vi "PathPlanner_ConstraintsZone_IsWithinZone.vi"(9 "T":dbl, 11 "ConstraintsZone":T1) -> (3 "WithinZone":bool)   [LabVIEW 2019, in "PathPlanner24.lvlib"]
doc: "Get if a given waypoint relative position is within this zone\n \nInputs:\n -- ConstraintsZone -- cluster -- data structure containing zone definition. \n -- t - double - Waypoint relative position\n\nOutputs:\n -- WithinZone - boolean - True if given position is within this zone"
uses:
  PathPlanner24.lvlib
  TypeDef/PathPlannerConstraintsZone.ctl
  TypeDef/PathPlannerPathConstraints.ctl
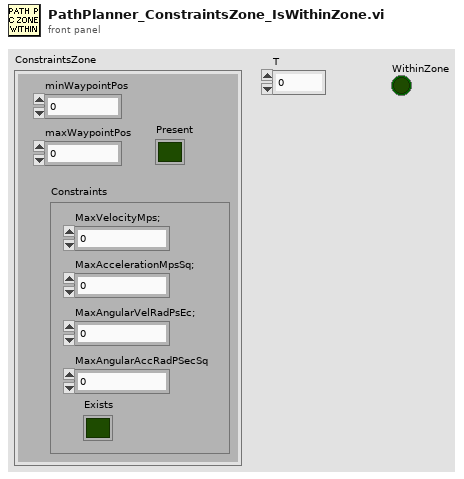
[diagram p1: front panel]
types:
  T1 = typedef "PathPlanner24.lvlib/PathPlannerConstraintsZone.ctl" = cluster{"minWaypointPos":dbl, "maxWaypointPos":dbl, "Constraints":T2, "Present":bool}
  T2 = typedef "PathPlanner24.lvlib/PathPlannerPathConstraints.ctl" = cluster{"MaxVelocityMps;":dbl, "MaxAccelerationMpsSq;":dbl, "MaxAngularVelRadPsEc;":dbl, "MaxAngularAccRadPSecSq":dbl, "Exists":bool}
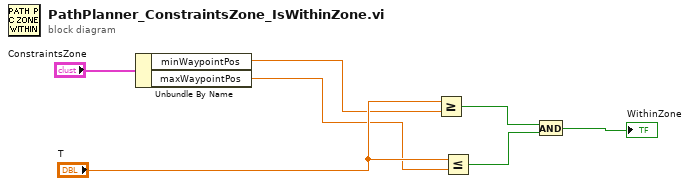
[diagram p0: block diagram]
diagram:
  n1 = Unbundle By Name("ConstraintsZone") -> ("minWaypointPos"=w5:dbl, "maxWaypointPos"=w4:dbl)
  n2 = Greater Or Equal?(x="T", y=w5) -> (x >= y?=w3:bool)
  n3 = Less Or Equal?(x="T", y=w4) -> (x <= y?=w2:bool)
  n4 = And(x=w3, y=w2) -> (x .and. y?=→"WithinZone":bool)
